vi "writeToXML.vi"(8 "error in (no error)":errorcluster, 10 "ClassLabel":string, 11 "GuideClear in":refnum<class "GuideClear.lvclass">) -> (0 "error out":errorcluster, 2 "XML out":string, 3 "GuideClear out":refnum<class "GuideClear.lvclass">)   [LabVIEW 2022 SP3, in "TCSDataDefinitions.lvlib" / "TCSCommand.lvlib" / "GuiderCommands.lvlib" / "GuideClear.lvclass"]
uses:
  GuideClear.lvclass
  GuiderCommands.lvclass
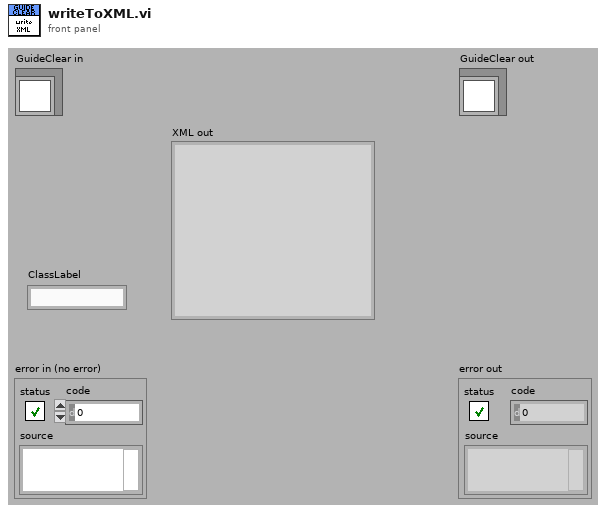
[diagram p1: front panel]
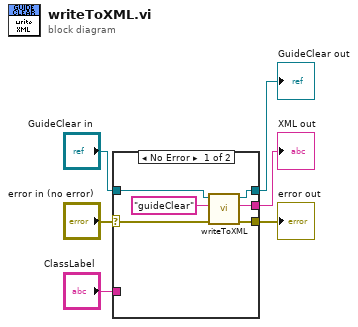
[diagram p0: block diagram]
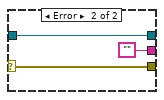
[diagram p2: hidden frame]
diagram:
  n1 = case shown="No Error" "error in (no error)" {
    selector: "error in (no error)" -> [w9 w15]
    tunnel: [w8 w15] -> w5
    tunnel: [w10 w14] -> w3
    tunnel: "GuideClear in" -> [w11 w14]
    tunnel: [w7 ""] -> w2
    tunnel: "ClassLabel" -> [_ _]
    frame No Error {
      n2 = call-parent "writeToXML.vi"("error in (no error)"=w9, "ClassLabel"="guideClear", "GuiderCommands in"=w11) -> ("error out"=w8:errorcluster, "XML out"=w7:string, "GuiderCommands out"=w10:refnum<class "GuideClear.lvclass">)  [unwired: 6 in]
    }
    frame Error {
    }
  }
  "error out" <- w5
  "GuideClear out" <- w3
  "XML out" <- w2
